vi "BSC top地址获取.vi"() -> ()   [LabVIEW 2020]
uses:
  <vilib>/httpClient/ClientHandle.ctl
  <vilib>/Utility/file.llb/Write Delimited Spreadsheet (string).vi
  <vilib>/httpClient/LabVIEWHTTPClient.lvlib
panel:
  in  "file path (dialog if empty)":path=path "D:/NI 资源包/2-币猎人-事件状态机930/source/网址私钥获取/btc搜寻器/BCS前10000账户.txt" caption="文件路径 （空时为对话框）"
  out "数组":string[][](array[string])
  out "添加的数组":string[](array[string])
  out "余额":string
  out "地址":string
  out "数组 2":string[](array[string])
  out "子字符串之前":string
  out "子字符串之后":string
  out "body":string caption="体部"
  out "headers":string caption="头部"
  out "error out":errorcluster caption="错误输出"
  in  "error in (no error)":errorcluster caption="错误输入（无错误）"
  in  "client handle":T1 caption="客户端句柄"
  out "URL输出":string
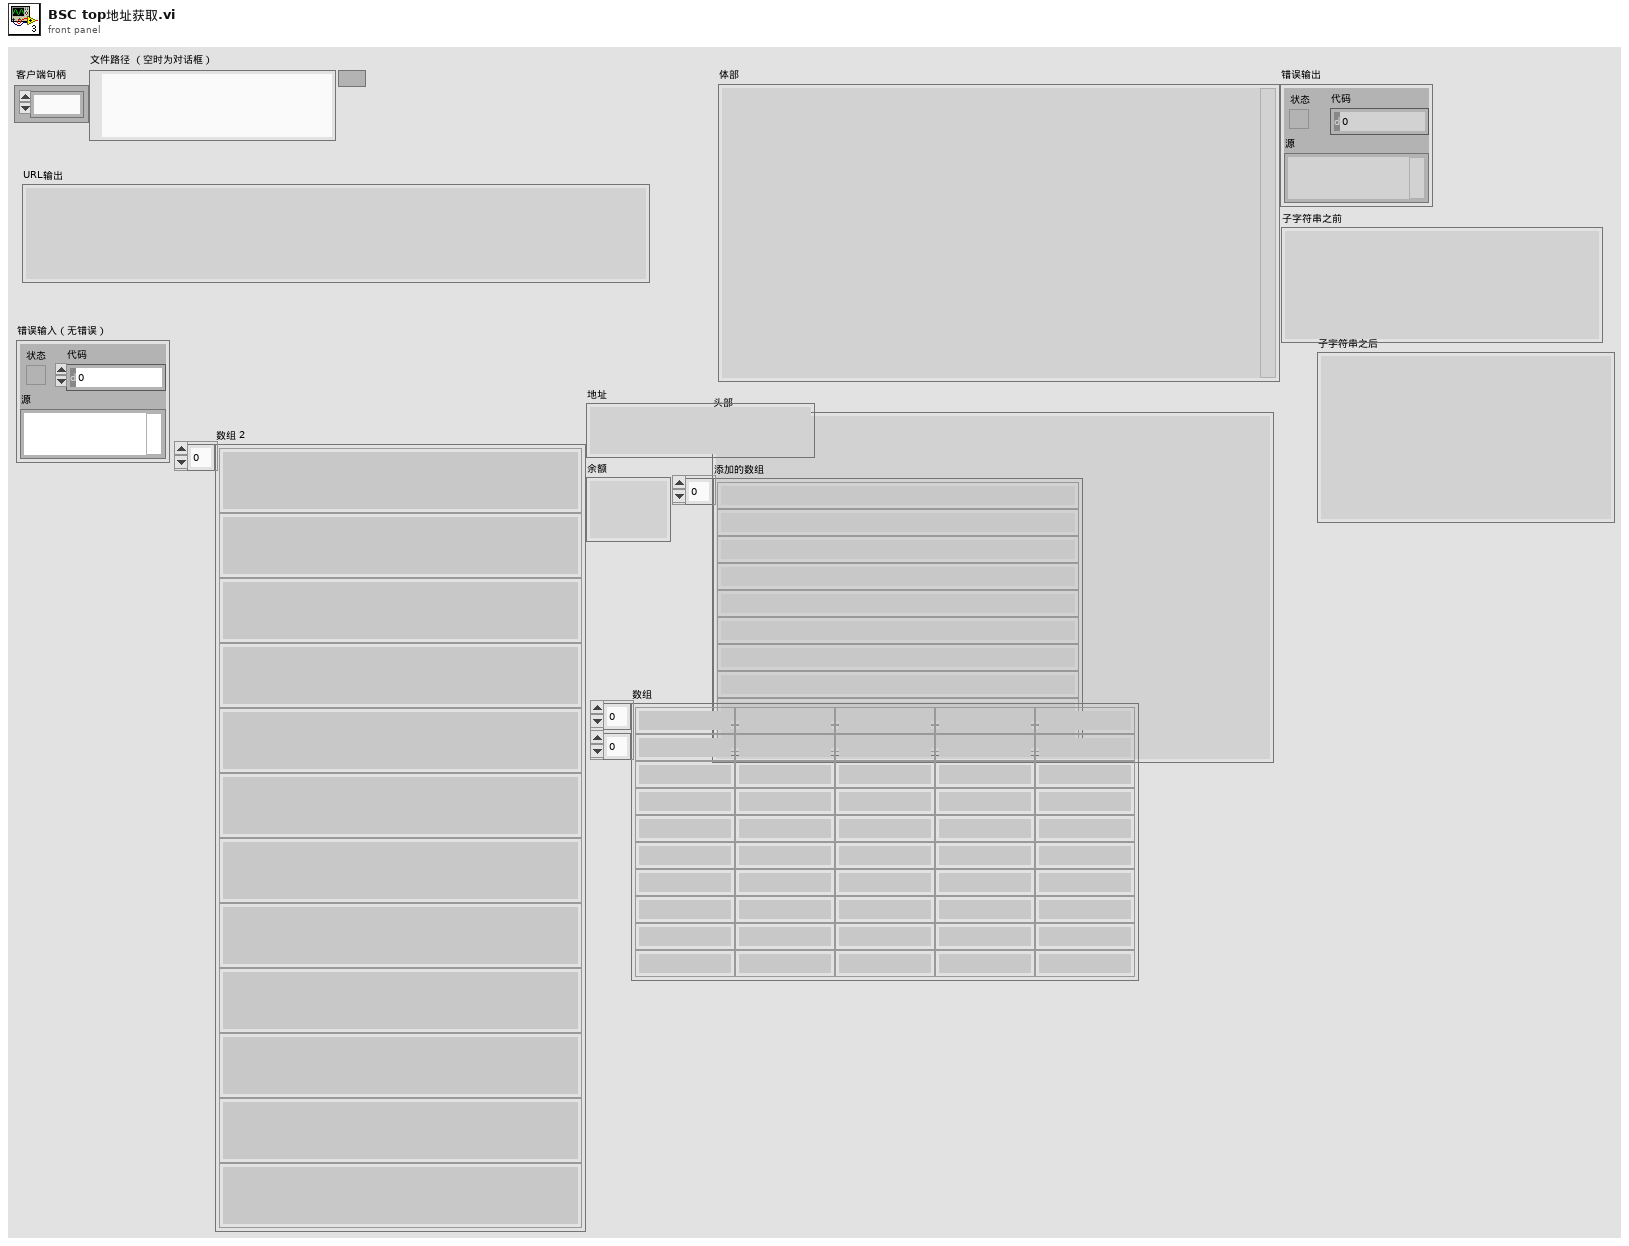
[diagram p1: front panel]
types:
  T1 = typedef "LabVIEWHTTPClient.lvlib/ClientHandle.ctl" = refnum<k1>
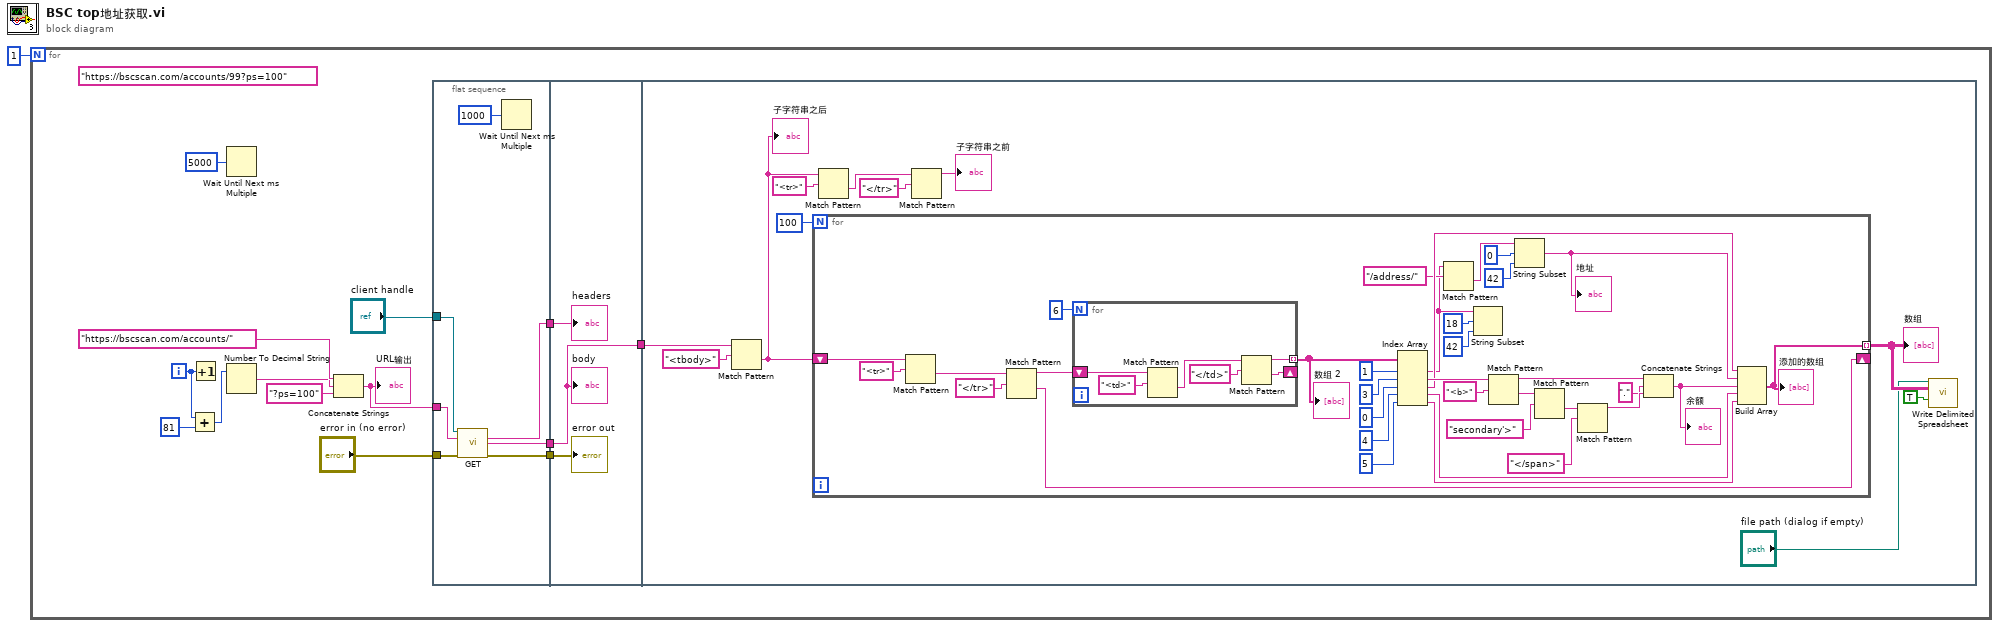
[diagram p0: block diagram]
diagram:
  n1 = for {
    N: 1 -> [_]
    i -> [w4]
    (unwired) "https://bscscan.com/accounts/99?ps=100" ("URL输入 2")
    n2 = Add(x=w4, y=81) -> (x+y=w2:i32)
    n3 = Increment(x=w4) -> ()  [unwired: 1 out]
    n4 = Wait Until Next ms Multiple(millisecond multiple=u32 5000 ("毫秒倍数")) -> ()  [unwired: 1 out]
    n5 = Number To Decimal String(number=w2) -> (decimal integer string=w8:string)  [unwired: 1 in]
    n6 = Concatenate Strings("https://bscscan.com/accounts/" ("URL输入 2"), w8, "?ps=100" ("字符串")) -> (w6:string)
    "URL输出" <- w6
    n7 = flat-sequence {
      tunnel: [w19] -> w15
      tunnel: [w18] -> w14
      tunnel: "client handle" -> [w22]
      tunnel: w6 -> [w21]
      tunnel: "error in (no error)" -> [w20]
      tunnel: [w16] -> w13
      tunnel: w15 -> [w25]
      tunnel: w14 -> [w23]
      tunnel: w13 -> [w24]
      tunnel: [w23] -> w12
      tunnel: w12 -> [w36]
      frame #0 {
        n8 = call <vilib>:"GET.vi"("client handle"=w22, "url"=w21, "error in (no error)"=w20) -> ("headers"=w19:string, "body"=w18:string, "error out"=w16:errorcluster)  [unwired: 9 in, 1 out]
        n9 = Wait Until Next ms Multiple(millisecond multiple=u32 1000 ("毫秒倍数")) -> ()  [unwired: 1 out]
      }
      frame #1 {
        "body" <- w23
        "headers" <- w25
        "error out" <- w24
      }
      frame #2 {
        n10 = Match Pattern(string=w36, regular expression="<tbody>") -> (after substring=w29:string)  [unwired: 1 in, 3 out]
        "子字符串之后" <- w29
        n11 = for {
          N: 100 -> [_]
          shift-right: [w67] -> _
          shift-left: w29 -> [w70]
          tunnel: [w43] -> w28 mode=indexing
          n12 = Match Pattern(string=w70, regular expression="<tr>") -> (after substring=w69:string)  [unwired: 1 in, 3 out]
          n13 = Match Pattern(string=w69, regular expression="</tr>" ("正则表达式")) -> (before substring=w44:string, after substring=w67:string)  [unwired: 1 in, 2 out]
          n14 = for {
            N: 6 -> [_]
            shift-right: [w73] -> _
            shift-left: w44 -> [w74]
            tunnel: [w72] -> w65 mode=indexing
            n15 = Match Pattern(string=w74, regular expression="<td>" ("正则表达式")) -> (after substring=w76:string)  [unwired: 1 in, 3 out]
            n16 = Match Pattern(string=w76, regular expression="</td>" ("正则表达式")) -> (before substring=w72:string, after substring=w73:string)  [unwired: 1 in, 2 out]
          }
          "数组 2" <- w65
          n17 = Index Array(array=w65, index #1=1 ("索引"), index #2=3 ("索引"), index #3=0 ("索引"), index #4=4 ("索引"), index #5=5 ("索引")) -> (element #1=w38:string, element #2=w60:string, element #3=w50:string, element #4=w46:string, element #5=w45:string)
          n18 = Match Pattern(string=w38, regular expression="/address/" ("正则表达式")) -> (after substring=w40:string)  [unwired: 1 in, 3 out]
          n19 = String Subset(string=w38, offset (0)=18 ("偏移量(0)"), length (rest)=42 ("长度（剩余）")) -> ()  [unwired: 1 out]
          n20 = Match Pattern(string=w60, regular expression="<b>" ("正则表达式")) -> (before substring=w54:string, after substring=w58:string)  [unwired: 1 in, 2 out]
          n21 = String Subset(string=w40, offset (0)=0 ("偏移量(0)"), length (rest)=42 ("长度（剩余）")) -> (substring=w37:string)
          "地址" <- w37
          n22 = Match Pattern(string=w58, regular expression="secondary'>" ("正则表达式")) -> (after substring=w56:string)  [unwired: 1 in, 3 out]
          n23 = Match Pattern(string=w56, regular expression="</span>" ("正则表达式")) -> (before substring=w53:string)  [unwired: 1 in, 3 out]
          n24 = Concatenate Strings(w54, "." ("字符串"), w53) -> (w49:string)
          "余额" <- w49
          n25 = Build Array(w50, w37, w49, w46, w45) -> (w43:string[])
          "添加的数组" <- w43
        }
        "数组" <- w28
        n26 = Match Pattern(string=w29, regular expression="<tr>") -> (after substring=w33:string)  [unwired: 1 in, 3 out]
        n27 = Match Pattern(string=w33, regular expression="</tr>" ("正则表达式")) -> (before substring=→"子字符串之前":string)  [unwired: 1 in, 3 out]
        n28 = call-poly <vilib>:"Write Delimited Spreadsheet.vi"("file path (dialog if empty)"="file path (dialog if empty)", "2D data"=w28, "append to file? (new file:F)"=TRUE) -> ()  [unwired: 11 in, 2 out]
      }
    }
  }
